vi "SetLibrarySDLPathIfSDL.vi"(8 "error in (no error)":errorcluster, 10 "Platform Type":T1, 11 "Library Call Ref":refnum<vi>) -> (0 "error out":errorcluster)   [LabVIEW 2024, in "Scripts.lvlib"]
uses:
  Scripts.lvlib
  PlatformType--enum.ctl
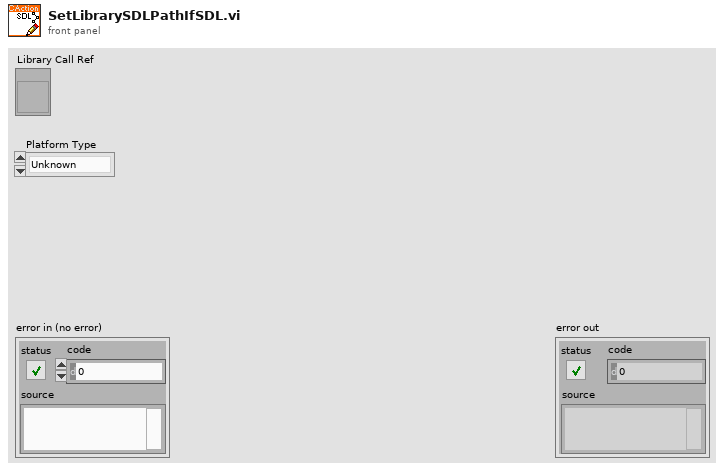
[diagram p1: front panel]
types:
  T1 = typedef "Scripts.lvlib/PlatformType--enum.ctl" = enum16{"Unknown", "Win32", "Win64", "Linux"}
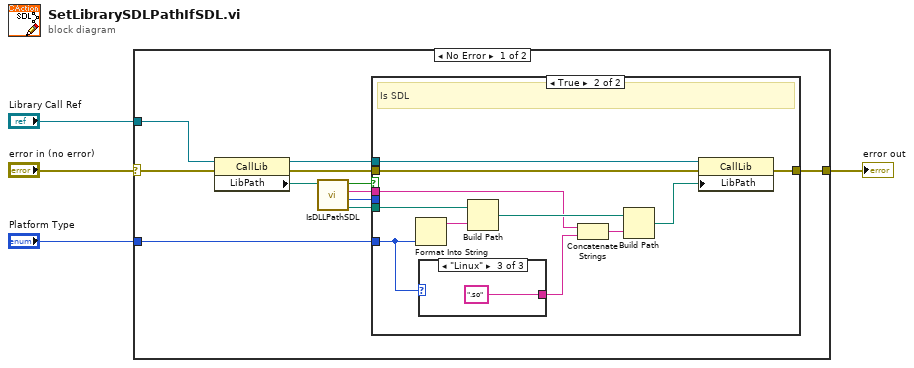
[diagram p0: block diagram]
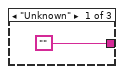
[diagram p3: hidden frame]
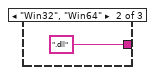
[diagram p4: hidden frame]
diagram:
  n1 = case shown="No Error" "error in (no error)" {
    selector: "error in (no error)" -> [w14 w31]
    tunnel: "Library Call Ref" -> [w15 _]
    tunnel: [w5 w31] -> w3
    tunnel: "Platform Type" -> [w6 _]
    frame No Error {
      n2 = property class="CallLib"(reference=w15, error in=w14) -> (reference out=w10:refnum<vi>, error out=w12:errorcluster, "LibPath"=w13:path)
      n3 = call "IsDLLPathSDL.vi"("DLL Path"=w13) -> ("Lib Folder"=w7:path, "Platform Type"=w8:T1, "Library Name"=w9:string, "Is SDL?"=w11:bool)  [unwired: 7 in]
      n4 = case shown="True" w11 {
        tunnel: w12 -> [w16 w27]
        tunnel: w10 -> [_ w25]
        tunnel: w9 -> [_ w21]
        tunnel: w8 -> [_ _]
        tunnel: w7 -> [_ w24]
        tunnel: w6 -> [_ w19]
        tunnel: [w16 w26] -> w5
        frame False {
          # "Not SDL"
        }
        frame True {
          # "Is SDL"
          n5 = Format Into String(w19) -> (resulting string=w23:string)  [unwired: 3 in, 1 out]
          n6 = case shown="\"Linux\"" w19 {
            tunnel: ["" ".dll" ".so"] -> w18
            frame "Unknown" {
            }
            frame "Win32", "Win64" {
            }
            frame "Linux" {
            }
          }
          n7 = Build Path(base path=w24, name or relative path=w23) -> (appended path=w22:path)
          n8 = Concatenate Strings(w21, w18) -> (w20:string)
          n9 = Build Path(base path=w22, name or relative path=w20) -> (appended path=w17:path)
          n10 = property class="CallLib"(reference=w25, error in=w27, "LibPath"=w17) -> (error out=w26:errorcluster)  [unwired: 1 out]
        }
      }
    }
    frame Error {
    }
  }
  "error out" <- w3
